vi "Teleop.vi"(10 "Match Info":T1={"Autonomous Elapsed Seconds"=0.0, "TeleOp Elapsed Seconds"=0.0, "Disabled Elapsed Seconds"=0.0, "Visited Autonomous"=FALSE, "Visited TeleOp"=FALSE, "Visited Disabled"=FALSE, "Autonomous Settings"={"Autonomous Style"=enum."Independent", "VI Refnum"=refnum}}, 11 "Call Context":T2) -> ()   [LabVIEW 2016]
doc: "This VI is called for each TeleOp packet received from the DS where the robot is not disabled. It is often used to read from the joysticks and update I/O or to update setpoints for timed control loops. It should complete and return within 20 milliseconds or it may miss DS packets."
uses:
  <vilib>/Rock Robotics/WPI/DriverStation/WPI_DriverStationDerivedRobotMode.ctl
  <vilib>/Rock Robotics/WPI/DriverStation/WPI_DriverStationMatch Info.ctl
  <vilib>/Rock Robotics/WPI/ThirdParty/CanMotor/TalonSRX/WPI_CANTalonSRX_APIFeedbackSelect.ctl
  <vilib>/Rock Robotics/WPI/ThirdParty/CanMotor/TalonSRX/WPI_CANTalonSRX_APIControlMode.ctl
  <vilib>/Rock Robotics/WPI/Utilities/WPI_GetSetVariantRefNum.vi
  <vilib>/Rock Robotics/Network Tables/NT Write Boolean Array.vi
  <vilib>/Rock Robotics/Network Tables/NT Write Numeric Array.vi
  <vilib>/Rock Robotics/Network Tables/NT Read Boolean.vi
  <vilib>/Rock Robotics/Network Tables/NT Read Number.vi
  Robot Global Data.vi
  <vilib>/Rock Robotics/Network Tables/NT Write Boolean.vi
panel:
  out "Value 2":bool
  out "Value":bool
  out "Left Encoder":dbl
  out "Right Encoder":dbl
  out "Battery Voltage":dbl
  out "Current":dbl
  out "SensorPosRotations":dbl
  out "Motor output Plot":cluster{"Applied Throttle":dbl}(graph)
  out "Target RPM":dbl
  out "SensorRPM Velocity RPM":dbl
  out "Applied Output":dbl
  out "Speed Closed Loop Plots":cluster{dbl, "Sensor Velocity":dbl}(graph)
  in  "Enable":bool=TRUE
  in  "Reset":bool
  out "Table":string[][](table)
  out "Encoder Velocity":dbl
  out "Sample Slider 0":dbl(slide) scale=0.0..5.0
  out "Sample Boolean 1":bool
  out "Sample Boolean 0":bool
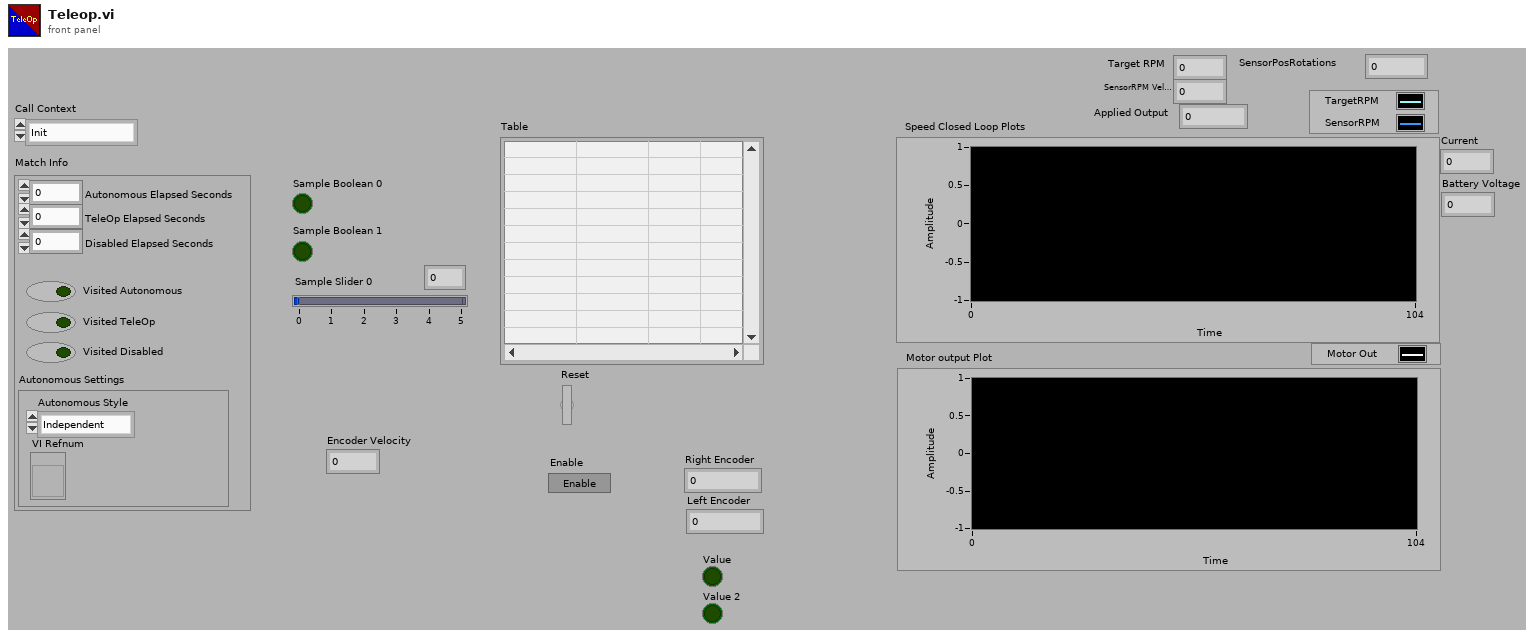
[diagram p1: front panel]
types:
  T1 = typedef "WPI_DriverStationMatch Info.ctl" = cluster{"Autonomous Elapsed Seconds":dbl, "TeleOp Elapsed Seconds":dbl, "Disabled Elapsed Seconds":dbl, "Visited Autonomous":bool, "Visited TeleOp":bool, "Visited Disabled":bool, "Autonomous Settings":cluster{"Autonomous Style":enum16{"Iterative", "Independent"}, "VI Refnum":refnum<vi>}}
  T2 = typedef "WPI_DriverStationDerivedRobotMode.ctl" = enum16{"Init", "Execute", "Stop"}
  T3 = typedef "WPI_CANTalonSRX_APIFeedbackSelect.ctl" = enum16{"Digital Quadrature Encoder", "Analog Potentiometer", "Analog Encoder", "Count on Quad-A (Rising-Edge)", "Count on Quad-A (Falling-Edge)", "CTR Magnetic Enc (Absolute)", "CTR Magnetic Enc (Relative)", "Pulse Width"}
  T4 = typedef "WPI_JoystickDevRef.ctl" = cluster{"Device":T5}
  T5 = typedef "WPI_JoystickDeviceEnum.ctl" = enum16{"USB 0", "USB 1", "USB 2", "USB 3", "USB 4", "USB 5"}
  T6 = typedef "WPI_RobotDriveDevRef.ctl" = cluster{"DevStatus":errorcluster, "Motors[]":T7[], "Square Inputs":bool, "Max Output":dbl}
  T7 = typedef "WPI_MotorControlDeviceRef.ctl" = cluster{"DeviceStatus":errorcluster, "Type":T8, "PWM":cluster{"PWM Channel":T9, "DeadBand":T10}, "CAN":cluster{"Device Number":u8, "SetOutput VI Ref":variant, "GetOutput VI Ref":variant, "Enable VI Ref":variant, "Disable VI Ref":variant, "Data":variant}, "Invert":bool}
  T8 = typedef "WPI_MotorControlType.ctl" = enum16{"PWM", "CAN"}
  T9 = typedef "FPGA_DIOPWMChannel.ctl" = enum8{"PWM 0", "PWM 1", "PWM 2", "PWM 3", "PWM 4", "PWM 5", "PWM 6", "PWM 7", "PWM 8", "PWM 9", "PWM MXP 0", "PWM MXP 1", "PWM MXP 2", "PWM MXP 3", "PWM MXP 4", "PWM MXP 5", "PWM MXP 6", "PWM MXP 7", "PWM MXP 8", "PWM MXP 9", "Invalid"}
  T10 = typedef "WPI_PWMDeadband.ctl" = cluster{"Name":string, "maxPositivePwm":i32, "minPositivePwm":i32, "centerPwm":i32, "maxNegativePwm":i32, "minNegativePwm":i32, "angularRange":u16}
  T11 = typedef "WPI_EncoderDevRef.ctl" = cluster{"DevStatus":errorcluster, "EncoderIndex":T12, "CounterIndex":T13, "DistancePerCount":dbl, "Decoding Type":T14}
  T12 = typedef "FPGA_EncoderIdx.ctl" = enum8{"Enc 0", "Enc 1", "Enc 2", "Enc 3", "Enc 4", "Enc 5", "Enc 6", "Enc 7", "Invalid"}
  T13 = typedef "FPGA_CounterCtrSystemIndex.ctl" = enum8{"Ctr 0", "Ctr 1", "Ctr 2", "Ctr 3", "Ctr 4", "Ctr 5", "Ctr 6", "Ctr 7", "Invalid"}
  T14 = typedef "WPI_EncoderType.ctl" = enum16{"1x", "2x", "4x"}
  T15 = typedef "WPI_CANTalonSRX_GlobalStatus.ctl" = cluster{"Applied Throttle":dbl, "Module Enabled":bool, "CAN Error":errorcluster, "Closed Loop Error":dbl, "Forward Limit Switch Closed":bool, "Reverse Limit Switch Closed":bool, "Sensor Position":dbl, "Sensor Velocity":dbl, "Current":dbl, "Sticky Fault - Over Temp":bool, "Sticky Fault - Under Voltage":bool, "Sticky Fault - Forward Limit":bool, "Sticky Fault - Reverse Limit":bool, "Sticky Fault - Forward Soft Limit":bool, "Sticky Fault - Reverse Soft Limit":bool, "Brake is Enabled":bool, "Encoder Position":dbl, "Encoder Velocity":dbl, "Encoder Index Count":dbl, "Encoder A Pin State":bool, "Encoder B Pin State":bool, "Encoder Index Pin State":bool, "Analog In":dbl, "Analog In Velocity":dbl, "Temperature (C)":dbl, "Battery Voltage":dbl, "Control 5 Is Supported":bool, "Current Profile Slot Select":dbl, "Pos Div 8":bool, "Vel Div 4":bool, "Pulse Width Position":i32, "Pulse Width Velocity":i32, "Pulse Width Rise To Rise (us)":i32, "Pulse Width Rise To Fall (us)":i32, "Mot Prof Active Is Under Run":bool, "Mot Prof Active Has Under Run":bool, "Mot Prof Active Is Last":bool, "Mot Prof Active Velocity Only":bool, "Mot Prof Active Is Valid":bool, "Mot Prof Buffer Is Full":bool, "Mot Prof Active Profile Slot Select":i32, "Mot Prof NextID":i32, "Mot Prof Count":i32, "Mot Prof Active Velocity":dbl, "Mot Prof Active Position":dbl, "Mot Prof Output Enable":i32, "UsageFrame":u32}
  T16 = typedef "WPI_DigitalInputDevRef.ctl" = cluster{"DevStatus":errorcluster, "DIO Channel":T17}
  T17 = typedef "FPGA_DIOChannel.ctl" = enum8{"DIO 0", "DIO 1", "DIO 2", "DIO 3", "DIO 4", "DIO 5", "DIO 6", "DIO 7", "DIO 8", "DIO 9", "DIO MXP 0", "DIO MXP 1", "DIO MXP 2", "DIO MXP 3", "DIO MXP 4", "DIO MXP 5", "DIO MXP 6", "DIO MXP 7", "DIO MXP 8", "DIO MXP 9", "DIO MXP 10", "DIO MXP 11", "DIO MXP 12", "DIO MXP 13", "DIO MXP 14", "DIO MXP 15", "SPI Port CS1", "SPI Port CS2", "SPI Port CS3", "SPI Port MISO", "SPI Port MOSI", "Invalid"}
  T18 = typedef "WPI_CANTalonSRX_APIControlMode.ctl" = enum8{"Percent VBus", "Speed", "Position", "Slave", "Unchanged / Invalid", "Voltage Compensation", "Current", "Motion Profile", "Motion Magic"}
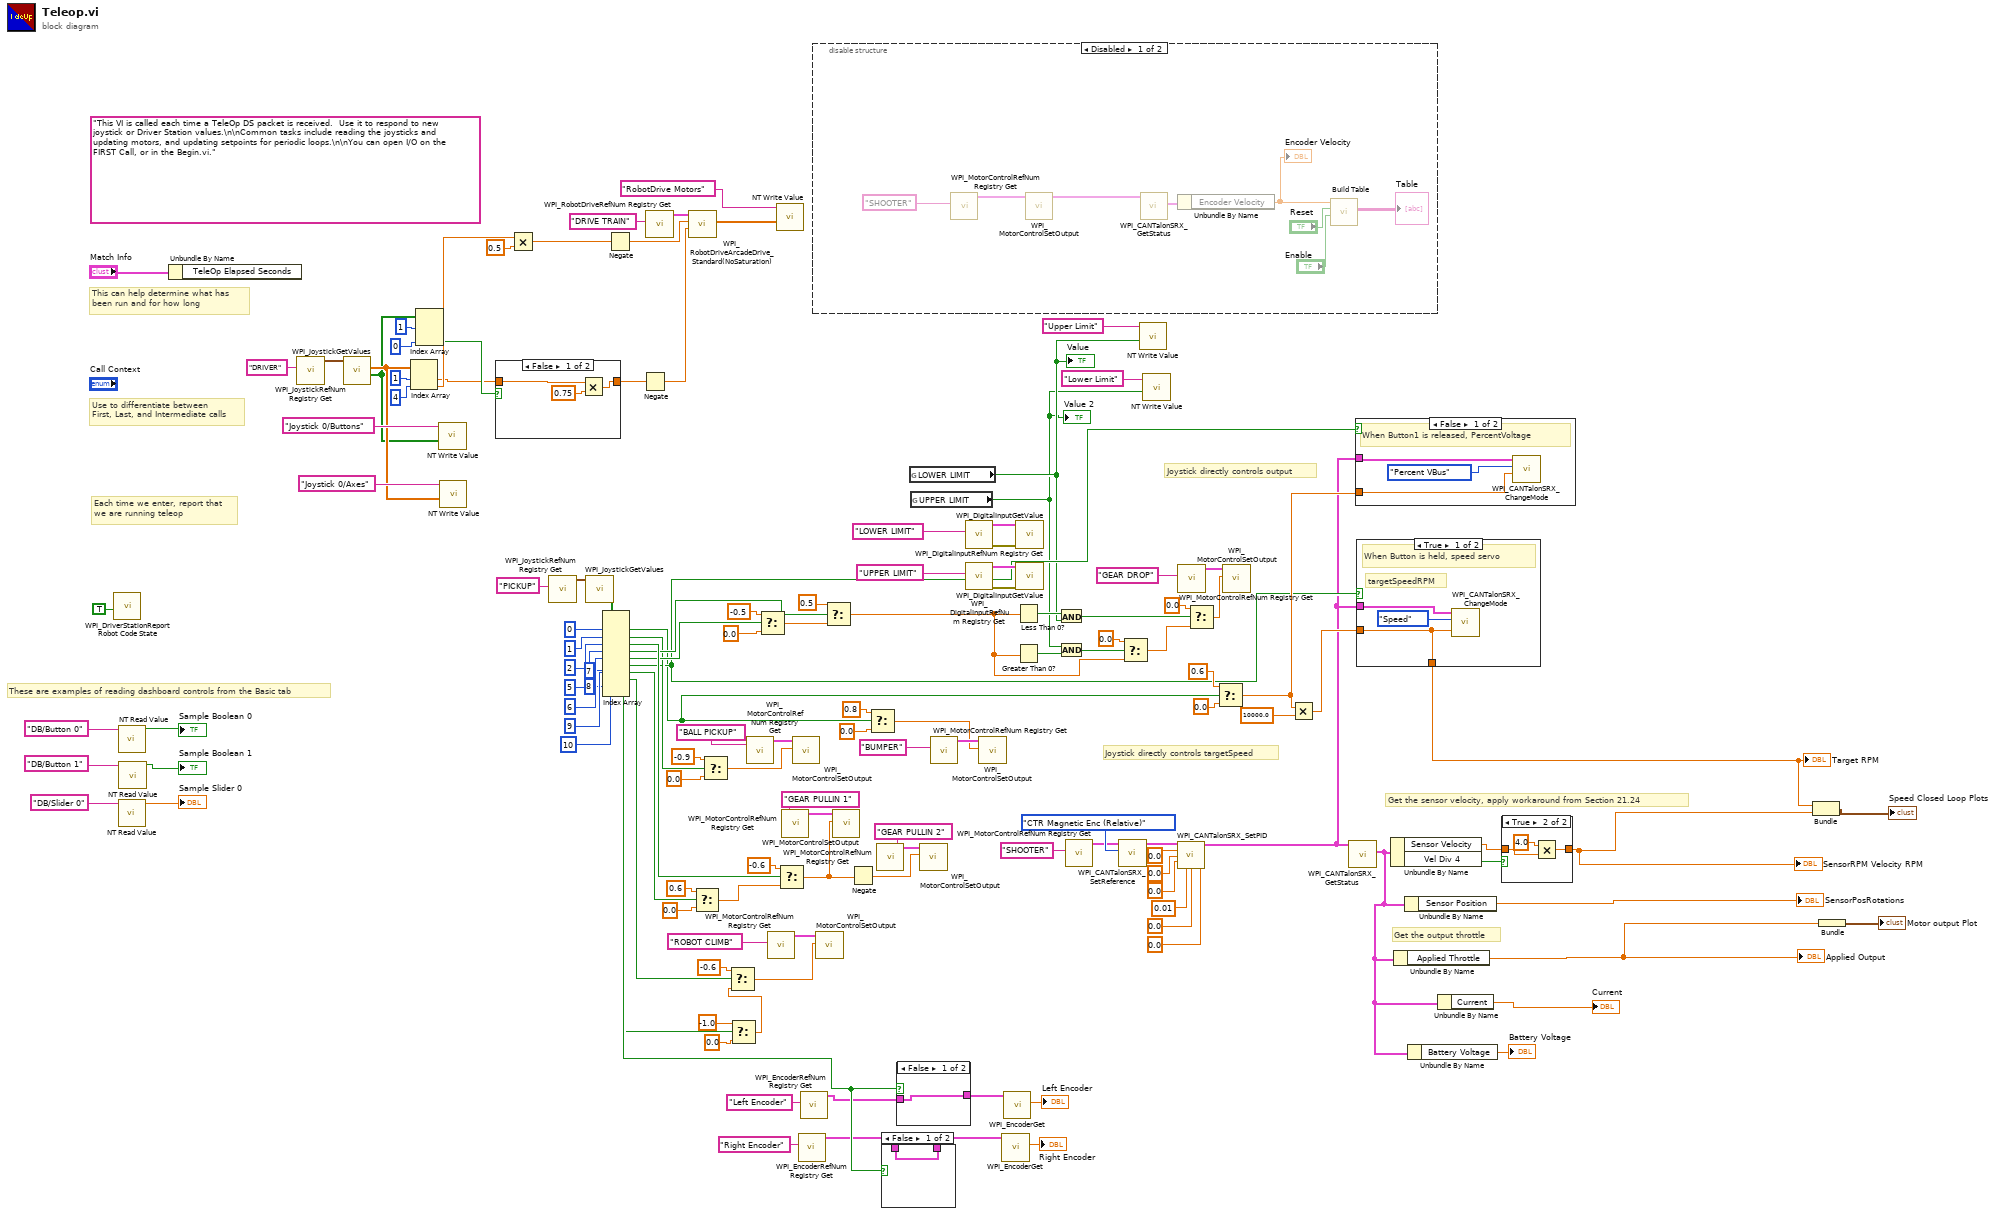
[diagram p0: block diagram]
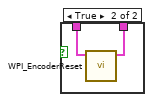
[diagram p2: hidden frame]
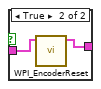
[diagram p3: hidden frame]
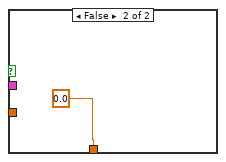
[diagram p8: hidden frame]
diagram:
  (unwired) "This VI is called each time a TeleOp DS packet is received.  Use it to respond to new joystick or Driver Station values.\n\nCommon tasks include reading the joysticks and updating motors, and updating setpoints for periodic loops.\n\nYou can open I/O on the FIRST Call, or in the Begin.vi."
  # "Get the output throttle"
  # "Get the sensor velocity, apply workaround from Section 21.24"
  # "Joystick directly controls targetSpeed"
  # "Joystick directly controls output"
  # "These are examples of reading dashboard controls from the Basic tab"
  # "Each time we enter, report that\nwe are running teleop"
  # "Use to differentiate between\nFirst, Last, and Intermediate calls"
  # "This can help determine what has\nbeen run and for how long"
  n1 = call <vilib>:"WPI_DriverStationReport Robot Code State.vi"("TeleOp"=TRUE ("Autonomous")) -> ()  [unwired: 10 in, 1 out]
  n2 = call-poly <vilib>:"NT Read Value.vi"("Name"="DB/Button 0" ("refnum name")) -> ("Boolean"=→"Sample Boolean 0":bool)  [unwired: 9 in, 1 out]
  n3 = call-poly <vilib>:"NT Read Value.vi"("Name"="DB/Slider 0" ("refnum name")) -> ("Numeric"=→"Sample Slider 0":dbl)  [unwired: 9 in, 1 out]
  n4 = call-poly <vilib>:"NT Read Value.vi"("Name"="DB/Button 1" ("refnum name")) -> ("Boolean"=→"Sample Boolean 1":bool)  [unwired: 9 in, 1 out]
  n5 = Unbundle By Name("Match Info") -> ()  [unwired: 1 out]
  n6 = call <vilib>:"WPI_JoystickRefNum Registry Get.vi"("refnum name"="DRIVER") -> ("JoystickDevRef"=w135:T4)  [unwired: 1 in, 9 out]
  n7 = call <vilib>:"WPI_JoystickGetValues.vi"("JoystickDevRef"=w135) -> ("Buttons"=w93:bool[], "Axes"=w131:dbl[])  [unwired: 6 in, 3 out]
  n8 = Index Array(array=w131, index #1=1 ("index"), index #2=4 ("index")) -> (element #1=w36:dbl, element #2=w89:dbl)
  n9 = Index Array(array=w93, index #1=1 ("index"), index #3=0 ("index")) -> (element #3=w37:bool)  [unwired: 1 in, 2 out]
  n10 = call-poly <vilib>:"NT Write Value.vi"("Boolean Array"=w93, "Name"="Joystick 0/Buttons") -> ()  [unwired: 9 in, 1 out]
  n11 = call-poly <vilib>:"NT Write Value.vi"("Numeric Array"=w131, "Name"="Joystick 0/Axes") -> ()  [unwired: 9 in, 1 out]
  n12 = case shown="False" w37 {
    tunnel: [w141 w143] -> w35
    tunnel: w36 -> [w140 w143]
    frame False {
      n13 = Multiply(x=w140, y=0.75) -> (x*y=w141:dbl)
    }
    frame True {
    }
  }
  n14 = Multiply(x=w89, y=0.5) -> (x*y=w80:dbl)
  n15 = call <vilib>:"WPI_JoystickRefNum Registry Get.vi"("refnum name"="PICKUP") -> ("JoystickDevRef"=w122:T4)  [unwired: 1 in, 9 out]
  n16 = call <vilib>:"WPI_JoystickGetValues.vi"("JoystickDevRef"=w122) -> ("Buttons"=w120:bool[])  [unwired: 6 in, 4 out]
  n17 = Index Array(array=w120, index #1=0 ("index"), index #2=1 ("index"), index #3=2 ("index"), index #4=5 ("index"), index #5=6 ("index"), index #7=9 ("index"), index #8=10 ("index"), index #9=8 ("index"), index #10=7 ("index")) -> (element #1=w45:bool, element #2=w96:bool, element #3=w103:bool, element #4=w102:bool, element #5=w101:bool, element #6=w48:bool, element #7=w31:bool, element #8=w20:bool, element #9=w10:bool, element #10=w4:bool)  [unwired: 1 in]
  n18 = Negate(x=w80) -> (-x=w79:dbl)
  n19 = Negate(x=w35) -> (-x=w81:dbl)
  n20 = call <vilib>:"WPI_RobotDriveRefNum Registry Get.vi"("refnum name"="DRIVE TRAIN") -> ("RobotDriveDevRef"=w137:T6)  [unwired: 1 in, 9 out]
  n21 = call <vilib>:"WPI_RobotDriveArcadeDrive_Standard(NoSaturation).vi"("Y axis value"=w81, "X axis value"=w79, "RobotDriveDevRef"=w137) -> ("Motor Values"=w124:dbl[])  [unwired: 1 in, 7 out]
  n22 = Select(t=0.6, s=w31, f=0.0) -> (s? t:f=w33:dbl)
  n23 = Select(t=-0.9, s=w96, f=0.0) -> (s? t:f=w98:dbl)
  n24 = Select(t=-1.0, s=w4, f=0.0) -> (s? t:f=w1:dbl)
  n25 = Select(t=-0.6, s=w20, f=w1) -> (s? t:f=w22:dbl)
  n26 = call <vilib>:"WPI_MotorControlRefNum Registry Get.vi"("refnum name"="BALL PICKUP") -> ("MotorControlDevRef"=w100:T7)  [unwired: 9 in, 1 out]
  n27 = Select(t=-0.5, s=w101, f=0.0) -> (s? t:f=w77:dbl)
  n28 = call <vilib>:"WPI_MotorControlRefNum Registry Get.vi"("refnum name"="ROBOT CLIMB") -> ("MotorControlDevRef"=w23:T7)  [unwired: 9 in, 1 out]
  n29 = call-poly <vilib>:"NT Write Value.vi"("Numeric Array"=w124, "Name"="RobotDrive Motors") -> ()  [unwired: 9 in, 1 out]
  n30 = Select(t=-0.6, s=w103, f=w33) -> (s? t:f=w113:dbl)
  n31 = call <vilib>:"WPI_MotorControlRefNum Registry Get.vi"("refnum name"="GEAR PULLIN 1") -> ("MotorControlDevRef"=w118:T7)  [unwired: 9 in, 1 out]
  n32 = call <vilib>:"WPI_MotorControlSetOutput.vi"("Output"=w98, "MotorControlDevRef"=w100) -> ()  [unwired: 7 in, 3 out]
  n33 = call <vilib>:"WPI_EncoderRefNum Registry Get.vi"("refnum name"="Right Encoder") -> ("EncoderDevRef"=w9:T11)  [unwired: 9 in, 1 out]
  n34 = call <vilib>:"WPI_EncoderRefNum Registry Get.vi"("refnum name"="Left Encoder") -> ("EncoderDevRef"=w7:T11)  [unwired: 9 in, 1 out]
  n35 = disable-structure shown="Disabled" {
    frame Disabled {
      n36 = call <vilib>:"WPI_MotorControlRefNum Registry Get.vi"("refnum name"="SHOOTER") -> ("MotorControlDevRef"=w144:T7)  [unwired: 9 in, 1 out]
      n37 = call <vilib>:"WPI_MotorControlSetOutput.vi"("MotorControlDevRef"=w144) -> ("MotorControlDevRef"=w151:T7)  [unwired: 8 in, 2 out]
      n38 = call <vilib>:"WPI_CANTalonSRX_GetStatus.vi"("CAN Talon SRX Ref"=w151) -> ("Talon SRX Status"=w150:T15)  [unwired: 8 in, 2 out]
      n39 = Unbundle By Name(w150) -> ("Encoder Velocity"=w148:dbl)
      "Encoder Velocity" <- w148
      n40 = call "Build Table"("Enable"="Enable", "Reset"="Reset", "Signals"=w148) -> ("Table"=→"Table":string[][])  [unwired: 2 in, 6 out]
    }
    frame Enabled {
    }
  }
  n41 = call <vilib>:"WPI_MotorControlSetOutput.vi"("Output"=w22, "MotorControlDevRef"=w23) -> ()  [unwired: 7 in, 3 out]
  n42 = Select(t=0.5, s=w102, f=w77) -> (s? t:f=w71:dbl)
  n43 = call <vilib>:"WPI_MotorControlSetOutput.vi"("Output"=w113, "MotorControlDevRef"=w118) -> ()  [unwired: 7 in, 3 out]
  n44 = Negate(x=w113) -> (-x=w112:dbl)
  n45 = Select(t=0.8, s=w45, f=0.0) -> (s? t:f=w42:dbl)
  n46 = call <vilib>:"WPI_MotorControlRefNum Registry Get.vi"("refnum name"="GEAR PULLIN 2") -> ("MotorControlDevRef"=w115:T7)  [unwired: 9 in, 1 out]
  n47 = case shown="False" w10 {
    tunnel: w9 -> [w152 w154]
    tunnel: [w152 w153] -> w8
    frame False {
    }
    frame True {
      n48 = call <vilib>:"WPI_EncoderReset.vi"("EncoderDevRef"=w154) -> ("EncoderDevRef"=w153:T11)  [unwired: 9 in, 1 out]
    }
  }
  n49 = case shown="False" w10 {
    tunnel: w7 -> [w155 w157]
    tunnel: [w155 w156] -> w6
    frame False {
    }
    frame True {
      n50 = call <vilib>:"WPI_EncoderReset.vi"("EncoderDevRef"=w157) -> ("EncoderDevRef"=w156:T11)  [unwired: 9 in, 1 out]
    }
  }
  n51 = global read "Robot Global Data.vi" "LOWER LIMIT"() -> (w13:bool)
  "Value" <- w13
  n52 = global read "Robot Global Data.vi" "UPPER LIMIT"() -> (w12:bool)
  "Value 2" <- w12
  n53 = call <vilib>:"WPI_MotorControlSetOutput.vi"("Output"=w112, "MotorControlDevRef"=w115) -> ()  [unwired: 7 in, 3 out]
  n54 = call <vilib>:"WPI_MotorControlRefNum Registry Get.vi"("refnum name"="BUMPER") -> ("MotorControlDevRef"=w47:T7)  [unwired: 9 in, 1 out]
  n55 = call <vilib>:"WPI_DigitalInputRefNum Registry Get.vi"("refnum name"="LOWER LIMIT") -> ("error out"=w84:errorcluster, "DigitalInputDevRef"=w85:T16)  [unwired: 9 in]
  n56 = call <vilib>:"WPI_DigitalInputRefNum Registry Get.vi"("refnum name"="UPPER LIMIT") -> ("error out"=w87:errorcluster, "DigitalInputDevRef"=w86:T16)  [unwired: 9 in]
  n57 = call <vilib>:"WPI_MotorControlSetOutput.vi"("Output"=w42, "MotorControlDevRef"=w47) -> ()  [unwired: 7 in, 3 out]
  n58 = call <vilib>:"WPI_EncoderGet.vi"("EncoderDevRef"=w8) -> ("Distance"=→"Right Encoder":dbl)  [unwired: 5 in, 5 out]
  n59 = call <vilib>:"WPI_EncoderGet.vi"("EncoderDevRef"=w6) -> ("Distance"=→"Left Encoder":dbl)  [unwired: 5 in, 5 out]
  n60 = Less Than 0?(x=w71) -> (x < 0?=w73:bool)
  n61 = Greater Than 0?(x=w71) -> (x > 0?=w74:bool)
  n62 = call <vilib>:"WPI_DigitalInputGetValue.vi"("error in (no error)"=w84, "DigitalInputDevRef"=w85) -> ()  [unwired: 7 in, 3 out]
  n63 = call <vilib>:"WPI_DigitalInputGetValue.vi"("error in (no error)"=w87, "DigitalInputDevRef"=w86) -> ()  [unwired: 7 in, 3 out]
  n64 = And(x=w73, y=w13) -> (x .and. y?=w75:bool)
  n65 = And(x=w12, y=w74) -> (x .and. y?=w76:bool)
  n66 = call <vilib>:"WPI_MotorControlRefNum Registry Get.vi"("refnum name"="SHOOTER") -> ("MotorControlDevRef"=w59:T7)  [unwired: 9 in, 1 out]
  n67 = call <vilib>:"WPI_CANTalonSRX_SetReference.vi"("Feedback Reference"=WPI_CANTalonSRX_APIFeedbackSelect."CTR Magnetic Enc (Relative)", "CAN Talon SRX Ref"=w59) -> ("CAN Talon SRX Ref"=w58:T7)  [unwired: 8 in, 1 out]
  n68 = Select(t=0.0, s=w76, f=w71) -> (s? t:f=w69:dbl)
  n69 = call-poly <vilib>:"NT Write Value.vi"("Boolean"=w13, "Name"="Upper Limit") -> ()  [unwired: 9 in, 1 out]
  n70 = call-poly <vilib>:"NT Write Value.vi"("Boolean"=w12, "Name"="Lower Limit") -> ()  [unwired: 9 in, 1 out]
  n71 = call <vilib>:"WPI_CANTalonSRX_SetPID.vi"("CAN Talon SRX Ref"=w58, "P"=0.0, "I"=0.0, "D"=0.0, "F"=0.01, "I Zone"=0.0, "Ramp Rate"=0.0) -> ("CAN Talon SRX Ref"=w29:T7)  [unwired: 7 in, 1 out]
  n72 = call <vilib>:"WPI_MotorControlRefNum Registry Get.vi"("refnum name"="GEAR DROP") -> ("MotorControlDevRef"=w110:T7)  [unwired: 9 in, 1 out]
  n73 = Select(t=0.0, s=w75, f=w69) -> (s? t:f=w78:dbl)
  n74 = Select(t=0.6 ("Output"), s=w45, f=0.0) -> (s? t:f=w50:dbl)
  n75 = call <vilib>:"WPI_MotorControlSetOutput.vi"("Output"=w78, "MotorControlDevRef"=w110) -> ()  [unwired: 7 in, 3 out]
  n76 = Multiply(x=w50, y=10000.0) -> (x*y=w53:dbl)
  n77 = call <vilib>:"WPI_CANTalonSRX_GetStatus.vi"("CAN Talon SRX Ref"=w29) -> ("Talon SRX Status"=w40:T15)  [unwired: 8 in, 2 out]
  n78 = case shown="False" w48 {
    tunnel: w29 -> [w159 _]
    tunnel: w50 -> [w158 _]
    frame False {
      # "When Button1 is released, PercentVoltage"
      n79 = call <vilib>:"WPI_CANTalonSRX_ChangeMode.vi"("Output"=w158, "Control Mode"=WPI_CANTalonSRX_APIControlMode."Percent VBus", "CAN Talon SRX Ref"=w159) -> ()  [unwired: 7 in, 2 out]
    }
    frame True {
    }
  }
  n80 = case shown="True" w48 {
    tunnel: w53 -> [w161 _]
    tunnel: w29 -> [w162 _]
    tunnel: [w161 0.0 ("x")] -> w52
    frame True {
      # "targetSpeedRPM"
      # "When Button is held, speed servo"
      n81 = call <vilib>:"WPI_CANTalonSRX_ChangeMode.vi"("Output"=w161, "Control Mode"=WPI_CANTalonSRX_APIControlMode."Speed", "CAN Talon SRX Ref"=w162) -> ()  [unwired: 7 in, 2 out]
    }
    frame False {
    }
  }
  "Target RPM" <- w52
  n82 = Unbundle By Name(w40) -> ("Sensor Velocity"=w62:dbl, "Vel Div 4"=w61:bool)
  n83 = Unbundle By Name(w40) -> ("Applied Throttle"=w54:dbl)
  "Applied Output" <- w54
  n84 = Unbundle By Name(w40) -> ("Sensor Position"=→"SensorPosRotations":dbl)
  n85 = Unbundle By Name(w40) -> ("Battery Voltage"=→"Battery Voltage":dbl)
  n86 = Unbundle By Name(w40) -> ("Current"=→"Current":dbl)
  n87 = case shown="True" w61 {
    tunnel: [w165 w167] -> w60
    tunnel: w62 -> [w165 w166]
    frame False {
    }
    frame True {
      n88 = Multiply(x=4.0, y=w166) -> (x*y=w167:dbl)
    }
  }
  "SensorRPM Velocity RPM" <- w60
  n89 = Bundle("x"=w52, "Sensor Velocity"=w60) -> (→"Speed Closed Loop Plots":cluster{"x":dbl, "Sensor Velocity":dbl})  [unwired: 1 in]
  n90 = Bundle("Applied Throttle"=w54) -> (→"Motor output Plot":cluster{"Applied Throttle":dbl})  [unwired: 1 in]
